vi "_io_read.vi"(4 "Simulation read buffer (\"Simulation\")":string="Simulation", 6 "Block Logging (F)":bool, 7 "Allow Assure End with LF":bool=TRUE, 8 "error in":errorcluster caption="error in (no error)", 10 "Max bytes to read (2048)":u32=2048, 11 "VISA resource name":refnum<visa-resource-name>) -> (0 "error out":errorcluster, 1 "Read bytes count":u32, 2 "Read buffer":string, 3 "VISA resource name out":refnum<visa-resource-name>)   [LabVIEW 2020, in "Rohde&Schwarz RTx Oscilloscopes.lvlib" / "rsidr_core.lvlib"]
uses:
  rsidr_core.lvlib
  type_Error_Codes.ctl
  _type_Operation_Fgv_Debug.ctl
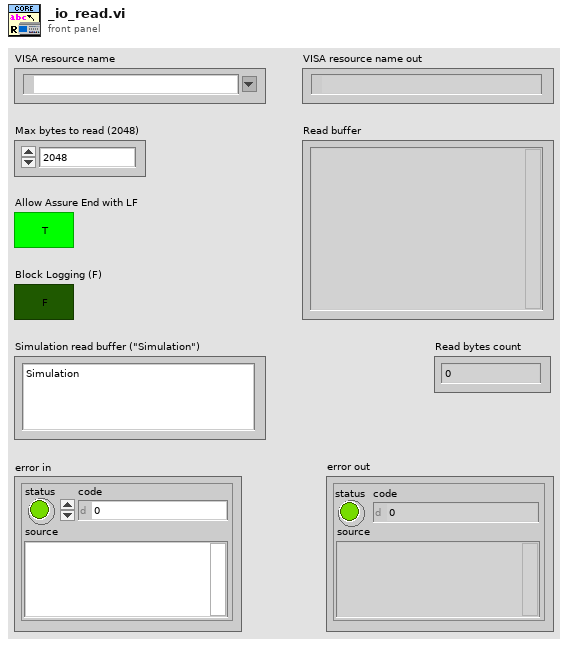
[diagram p1: front panel]
types:
  T1 = typedef "Rohde&Schwarz RTx Oscilloscopes.lvlib/rsidr_core.lvlib/_type_Operation_Fgv_Debug.ctl" = enum16{"Reset", "ReadCommand", "SetCommand"}
  T2 = typedef "Rohde&Schwarz RTx Oscilloscopes.lvlib/rsidr_core.lvlib/type_Session_Data.ctl" = cluster{"IDN string":string, "Instrument FW":string, "Instr type":string, "Instr type for err. msg.":string, "Installed Options":string[], "Ignore Error Messages":string, "Logging params":variant, "OPC Timeout":i32, "VISA Timeout":i32, "STB Poll VISA Timeout":i32, "Additional Flags":i32, "Wait Before Read":i32, "Wait Before Write":i32, "Option String Flags":i32, "IO Segment Size":i64, "VISA Access Mode":T3, "Interface Type":T4, "OPC Wait Mode":T5, "Bin Float Number  Format":T6, "Bin Integer Number Format":T7, "Simulate":bool, "VXIcapable":bool, "Duplicate Session":bool, "Add LF to Write":bool, "Logging":bool, "Fast Sweep":bool, "Query Instrument Status":bool, "Check Range":bool, "Check Options":bool, "OPC-sync Attr Writes":bool, "OPC-sync Attr Queries":bool}
  T3 = typedef "Rohde&Schwarz RTx Oscilloscopes.lvlib/rsidr_core.lvlib/type_VisaAccessMode.ctl" = u16
  T4 = typedef "Rohde&Schwarz RTx Oscilloscopes.lvlib/rsidr_core.lvlib/type_InterfaceType.ctl" = enum16{"Unknown", "GPIB", "VXI", "GPIB_VXI", "ASRL", "PXI", "TCPIP", "USB", "SOCKET"}
  T5 = typedef "Rohde&Schwarz RTx Oscilloscopes.lvlib/rsidr_core.lvlib/type_OPC_Wait_Mode.ctl" = enum16{"STBpolling", "STBpollingSlow", "STBpollingSuperSlow", "ServiceRequest", "OPCquery"}
  T6 = typedef "Rohde&Schwarz RTx Oscilloscopes.lvlib/rsidr_core.lvlib/type_Binary_Float_Number_Format.ctl" = enum16{"Float_4_Bytes_Swapped", "Float_4_Bytes", "Double_8_Bytes_Swapped", "Double_8_Bytes"}
  T7 = typedef "Rohde&Schwarz RTx Oscilloscopes.lvlib/rsidr_core.lvlib/type_Binary_Integer_Number_Format.ctl" = enum16{"Int32_4_Bytes_Swapped", "Int32_4 Bytes", "Int16_2_Bytes_Swapped", "Int16_2_Bytes"}
  T8 = typedef "Rohde&Schwarz RTx Oscilloscopes.lvlib/rsidr_core.lvlib/type_Error_Codes.ctl" = enum16{"No_error", "VISA_err_ResourceNotFound", "VISA_err_Timeout", "VISA_warn_MoreDataAvailable", "RS_err_MissingCallback", "RS_err_InvalidAttribute", "RS_err_InvalidValue", "RS_err_UnknownResource", "RS_err_AlreadyInitialized", "RS_err_InstrumentStatus", "RS_err_BadRepCapName", "RS_err_TypesMismatch", "RS_err_ValueNotSupported", "RS_err_InvalidRngTable", "RS_err_IDqueryFail", "RS_err_UnexpResponse", "VISA_warn_ConfigNotLoaded", "RS_err_AttributeNotReadable", "RS_err_AttributeNotWritable", "RS_err_InstrumentType", "RS_err_InstrumentOption", "VISA_err_InvalidSize", "RS_err_ReliabilityIndicator", "VISA_warn_UnknownStatus", "VISA_warn_TermCharRead", "VISA_err_IO_error", "RS_err_FunctionNotSupported", "VISA_warn_QueueEmpty"}
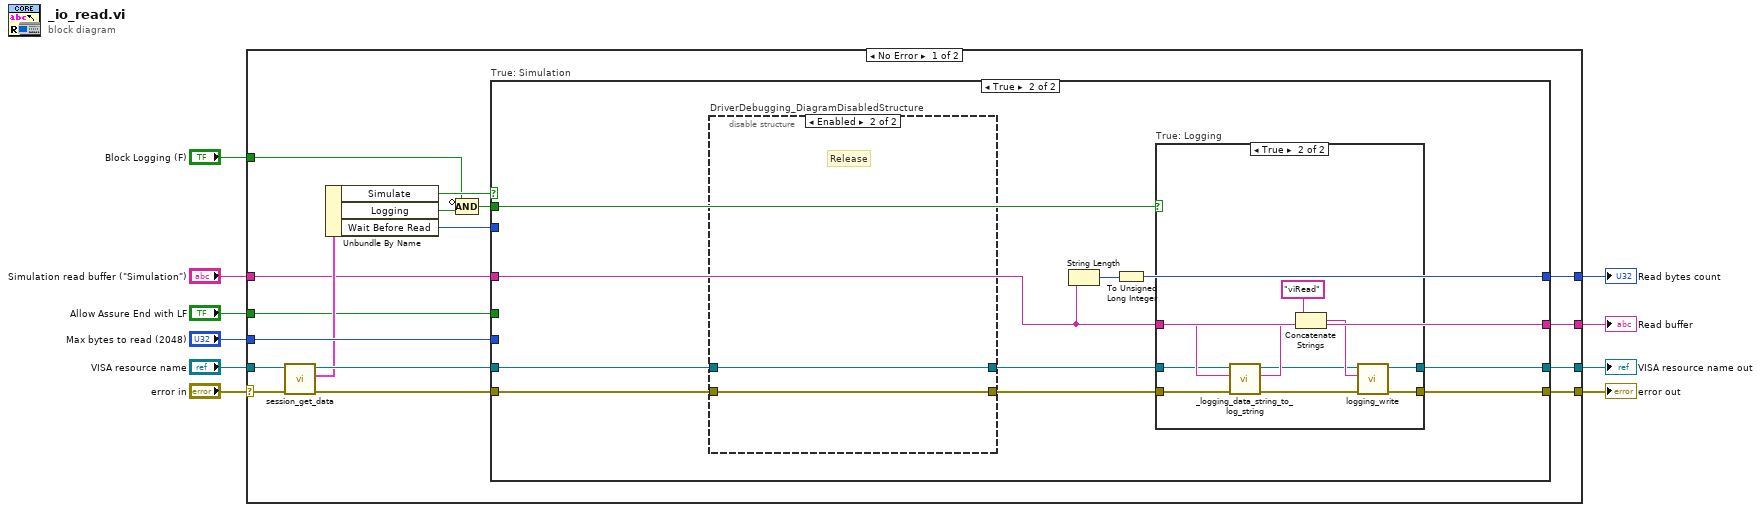
[diagram p0: block diagram]
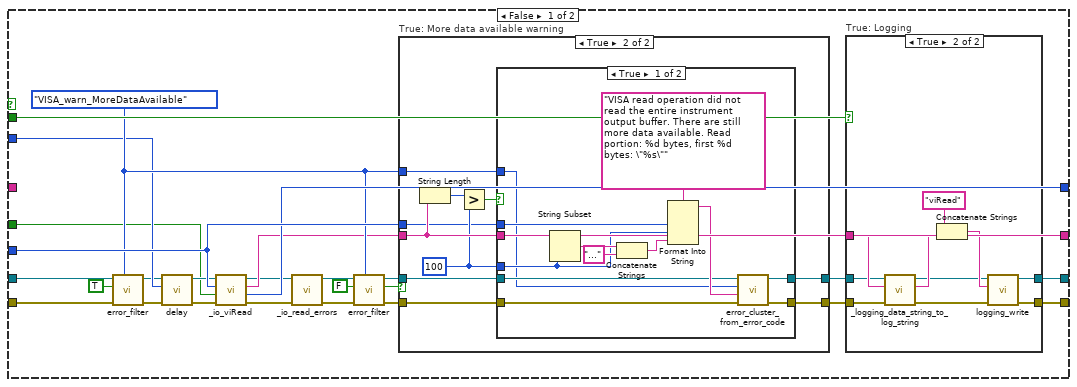
[diagram p2: hidden frame]
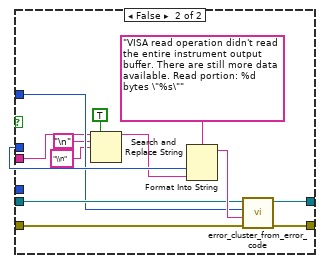
[diagram p5: hidden frame]
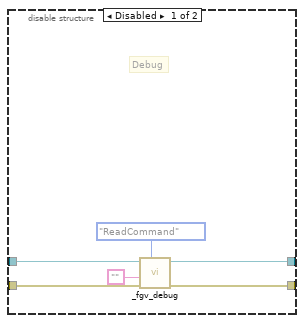
[diagram p6: hidden frame]
diagram:
  n1 = case shown="No Error" "error in" {
    selector: "error in" -> [w24 w135]
    tunnel: [w18 w135] -> w7
    tunnel: "Max bytes to read (2048)" -> [w27 _]
    tunnel: [w26 _] -> w9
    tunnel: "VISA resource name" -> [w23 w134]
    tunnel: [w25 _] -> w8
    tunnel: [w17 w134] -> w6
    tunnel: "Block Logging (F)" -> [w13 _]
    tunnel: "Simulation read buffer (\"Simulation\")" -> [w12 _]
    tunnel: "Allow Assure End with LF" -> [w11 _]
    frame No Error {
      n2 = call "session_get_data.vi"("error in"=w24, "VISA resource name"=w23) -> ("error out"=w22:errorcluster, "Session User Data out"=w20:T2, "VISA resource name out"=w21:refnum<visa-resource-name>)  [unwired: 6 in, 1 out]
      n3 = Unbundle By Name(w20) -> ("Simulate"=w19:bool, "Logging"=w16:bool, "Wait Before Read"=w14:i32)
      n4 = Compound Arithmetic op=AND(invert w13, w16) -> (w15:bool)
      n5 = case "True: Simulation" shown="True" w19 {
        tunnel: [w53 w111] -> w18
        tunnel: w27 -> [w52 _]
        tunnel: [w31 w104] -> w26
        tunnel: [w43 w109] -> w25
        tunnel: w22 -> [w42 w108]
        tunnel: w21 -> [w35 w106]
        tunnel: w15 -> [w50 w112]
        tunnel: [w51 w110] -> w17
        tunnel: w14 -> [w36 _]
        tunnel: w12 -> [_ w104]
        tunnel: w11 -> [w28 _]
        frame False {
          w41 = type_Error_Codes."VISA_warn_MoreDataAvailable" ("Code to detect")
          n6 = call "error_filter.vi"("Error Enum in"=w41, "error in"=w42, "Clear detected code (F)"=TRUE, "VISA resource name"=w35) -> ("error out"=w39:errorcluster, "VISA resource name out"=w34:refnum<visa-resource-name>)  [unwired: 5 in, 1 out]
          n7 = call "delay.vi"("error in"=w39, "Milliseconds to wait"=w36, "VISA resource name"=w34) -> ("error out"=w38:errorcluster, "VISA resource name out"=w37:refnum<visa-resource-name>)  [unwired: 7 in]
          n8 = call "_io_viRead.vi"("error in"=w38, "Allow Assure End with LF"=w28, "Max bytes to read"=w52, "VISA resource name"=w37) -> ("error out"=w29:errorcluster, "Read bytes count"=w43:u32, "Read buffer"=w31:string, "VISA resource name out"=w30:refnum<visa-resource-name>)  [unwired: 4 in]
          n9 = call "_io_read_errors.vi"("error in"=w29, "VISA resource name"=w30) -> ("error out"=w44:errorcluster, "VISA resource name out"=w33:refnum<visa-resource-name>)  [unwired: 8 in]
          n10 = call "error_filter.vi"("Error Enum in"=w41, "error in"=w44, "Clear detected code (F)"=FALSE ("Clear detected error (F)"), "VISA resource name"=w33) -> ("error out"=w48:errorcluster, "Code Detected"=w47:bool, "VISA resource name out"=w32:refnum<visa-resource-name>)  [unwired: 5 in]
          n11 = case "True: More data available warning" shown="True" w47 {
            tunnel: w48 -> [w67 w73]
            tunnel: [w67 w72] -> w46
            tunnel: w31 -> [_ w77]
            tunnel: w52 -> [_ w71]
            tunnel: w41 -> [_ w70]
            tunnel: w32 -> [w66 w69]
            tunnel: [w66 w68] -> w45
            frame False {
            }
            frame True {
              w75 = 100 ("length (rest)")
              n12 = String Length(string=w77) -> (length=w76:i32)
              n13 = Greater?(x=w76, y=w75) -> (0:w74:bool)
              n14 = case shown="True" w74 {
                tunnel: w77 -> [w90 w95]
                tunnel: w75 -> [w82 _]
                tunnel: w73 -> [w87 w103]
                tunnel: [w86 w102] -> w72
                tunnel: w71 -> [w84 w100]
                tunnel: w70 -> [w79 w96]
                tunnel: w69 -> [w81 w97]
                tunnel: [w80 w99] -> w68
                frame True {
                  n15 = String Subset(string=w90, length (rest)=w82) -> (substring=w89:string)  [unwired: 1 in]
                  n16 = Concatenate Strings(w89, "...") -> (w78:string)
                  n17 = Format Into String(format string="VISA read operation did not read the entire instrument output buffer. There are still more data available. Read portion: %d bytes, first %d bytes: \"%s\"", w84, w82, w78) -> (resulting string=w83:string)  [unwired: 2 in, 1 out]
                  n18 = call "error_cluster_from_error_code.vi"("error in"=w87, "Error Message (\"\")"=w83, "Error Enum in"=w79, "VISA resource name"=w81) -> ("error out"=w86:errorcluster, "VISA resource name out"=w80:refnum<visa-resource-name>)  [unwired: 6 in]
                }
                frame False {
                  n19 = Search and Replace String(replace all?=TRUE ("replace all? (F)"), input string=w95, search string="\n" ("Line Feed Constant"), replace string="\\n") -> (result string=w91:string)  [unwired: 4 in, 3 out]
                  n20 = Format Into String(format string="VISA read operation didn't read the entire instrument output buffer. There are still more data available. Read portion: %d bytes \"%s\"", w100, w91) -> (resulting string=w98:string)  [unwired: 2 in, 1 out]
                  n21 = call "error_cluster_from_error_code.vi"("error in"=w103, "Error Message (\"\")"=w98, "Error Enum in"=w96, "VISA resource name"=w97) -> ("error out"=w102:errorcluster, "VISA resource name out"=w99:refnum<visa-resource-name>)  [unwired: 6 in]
                }
              }
            }
          }
          n22 = case "True: Logging" shown="True" w50 {
            tunnel: w46 -> [w55 w59]
            tunnel: [w54 w65] -> w51
            tunnel: [w55 w64] -> w53
            tunnel: w31 -> [_ w63]
            tunnel: w45 -> [w54 w58]
            frame False {
            }
            frame True {
              n23 = call "_logging_data_string_to_log_string.vi"("error in"=w59, "Raw string to log"=w63, "VISA resource name"=w58) -> ("error out"=w57:errorcluster, "Result log string"=w61:string, "VISA resource name out"=w56:refnum<visa-resource-name>)  [unwired: 6 in]
              n24 = Concatenate Strings("viRead" ("format string"), w61) -> (w60:string)
              n25 = call "logging_write.vi"("error in"=w57, "String to write"=w60, "VISA resource name"=w56) -> ("error out"=w64:errorcluster, "VISA resource name out"=w65:refnum<visa-resource-name>)  [unwired: 7 in]
            }
          }
        }
        frame True {
          n26 = disable-structure "DriverDebugging_DiagramDisabledStructure" shown="Enabled" {
            disable-tunnel: w108 -> [w119 w120]
            disable-tunnel: [w117 w120] -> w107
            disable-tunnel: w106 -> [w118 w121]
            disable-tunnel: [w116 w121] -> w105
            frame Disabled {
              # "Debug"
              n27 = call "_fgv_debug.vi"("Operation"=_type_Operation_Fgv_Debug."ReadCommand", "error in"=w119, "Command in"="" ("Empty String Constant"), "VISA resource name"=w118) -> ("error out"=w117:errorcluster, "VISA resource name out"=w116:refnum<visa-resource-name>)  [unwired: 6 in]
            }
            frame Enabled {
              # "Release"
            }
          }
          n28 = String Length(string=w104) -> (length=w113:i32)
          n29 = To Unsigned Long Integer(number=w113) -> (unsigned 32bit integer=w109:u32)
          n30 = case "True: Logging" shown="True" w112 {
            tunnel: w104 -> [_ w131]
            tunnel: w107 -> [w123 w127]
            tunnel: w105 -> [w122 w126]
            tunnel: [w123 w133] -> w111
            tunnel: [w122 w132] -> w110
            frame False {
            }
            frame True {
              n31 = call "_logging_data_string_to_log_string.vi"("error in"=w127, "Raw string to log"=w131, "VISA resource name"=w126) -> ("error out"=w125:errorcluster, "Result log string"=w130:string, "VISA resource name out"=w124:refnum<visa-resource-name>)  [unwired: 6 in]
              n32 = Concatenate Strings("viRead" ("format string"), w130) -> (w129:string)
              n33 = call "logging_write.vi"("error in"=w125, "String to write"=w129, "VISA resource name"=w124) -> ("error out"=w133:errorcluster, "VISA resource name out"=w132:refnum<visa-resource-name>)  [unwired: 7 in]
            }
          }
        }
      }
    }
    frame Error {
    }
  }
  "VISA resource name out" <- w6
  "error out" <- w7
  "Read buffer" <- w9
  "Read bytes count" <- w8
